vi "QueueLV2G.vi"(0 "r":cluster{"h":dbl, "l":dbl, "c":dbl, "s":bool}, 11 "error in (no error)":errorcluster, 12 "Selector":T1(ring)) -> (4 "r[]":cluster{"h":dbl, "l":dbl, "c":dbl, "s":bool}[](array[cluster]), 15 "error out":errorcluster)   [LabVIEW 2016, in "Data Library.lvlib"]
uses:
  Data Library.lvlib
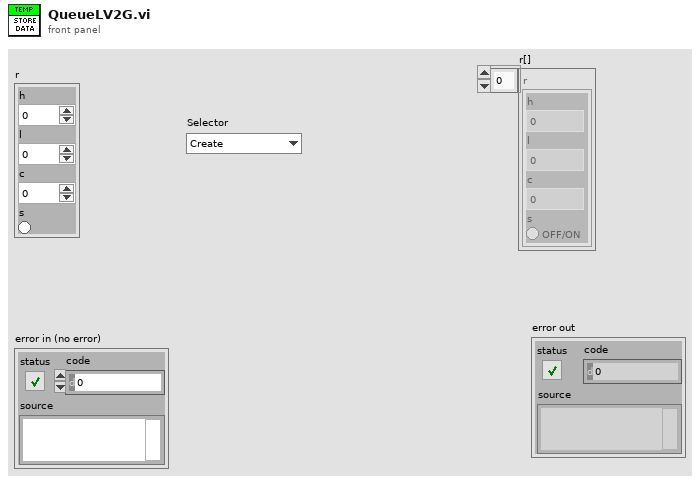
[diagram p1: front panel]
types:
  T1 = enum16{"Create", "Enqueue", "Preview Data", "Destroy"}
  T2 = cluster{"High Set Point":dbl, "Low Set Point":dbl, "Current Temperature":dbl, "Heater State?":bool}[]
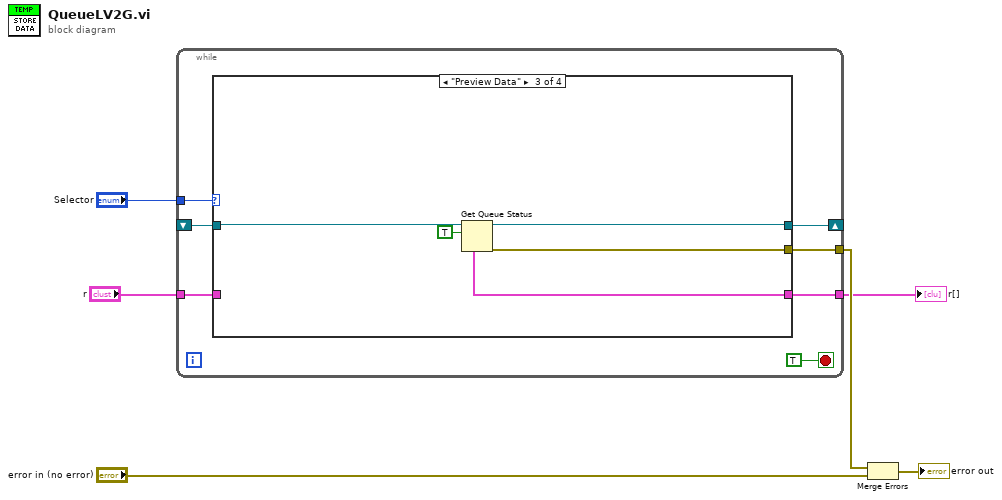
[diagram p0: block diagram]
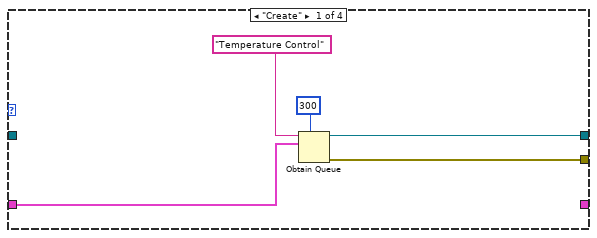
[diagram p2: hidden frame]
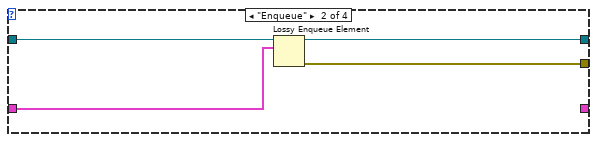
[diagram p3: hidden frame]
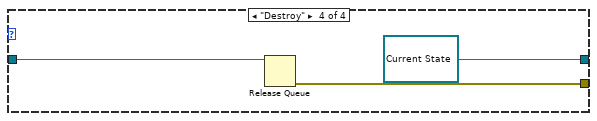
[diagram p4: hidden frame]
diagram:
  n1 = while {
    tunnel: "Selector" -> [w12]
    shift-right: [w11] -> _
    shift-left: _ -> [w9]
    tunnel: [w10] -> w5
    tunnel: "r" -> [w8]
    tunnel: [w7] -> w1
    stop <- TRUE stop-if-true
    n2 = case shown="\"Preview Data\"" w12 {
      tunnel: [w18 w21 w26 refnum<queue> refnum ("queue out")] -> w11
      tunnel: [w17 w20 w25 w29] -> w10
      tunnel: w9 -> [_ w22 w27 w30]
      tunnel: w8 -> [w15 w19 _ _]
      tunnel: [_ _ w24 _] -> w7
      frame "Create" {
        n3 = Obtain Queue(max queue size (-1, unlimited)=300, name (unnamed)="Temperature Control", element data type=w15) -> (queue out=w18:refnum<queue>, error out=w17:errorcluster)  [unwired: 2 in, 1 out]
      }
      frame "Enqueue" {
        n4 = Lossy Enqueue Element(queue=w22, element=w19) -> (queue out=w21:refnum<queue>, error out=w20:errorcluster)  [unwired: 1 in, 2 out]
      }
      frame "Preview Data" {
        n5 = Get Queue Status(queue=w27, return elements? (F)=TRUE) -> (queue out=w26:refnum<queue>, error out=w25:errorcluster, elements=w24:T2)  [unwired: 1 in, 5 out]
      }
      frame "Destroy" {
        n6 = Release Queue(queue=w30) -> (error out=w29:errorcluster)  [unwired: 2 in, 2 out]
      }
    }
  }
  "r[]" <- w1
  n7 = Merge Errors(w5, "error in (no error)") -> (→"error out":errorcluster)
